vi "Parse Floating Point String As Extended.vi"(8 "error in (no error)":errorcluster, 11 "String":string) -> (0 "error out":errorcluster, 3 "Value":variant)   [LabVIEW 2019, in "JKI JSON Serialization.lvlib" / "JSON Parser.lvclass"]
doc: "JKI JSON 1.1.10.37\nTomi Maila - JKI\nCopyright (c) 2017, JKI"
uses:
  JSON Parser.lvclass
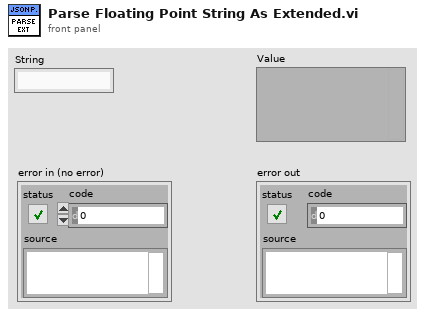
[diagram p1: front panel]
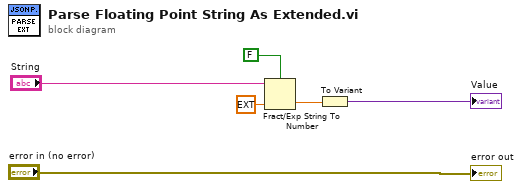
[diagram p0: block diagram]
diagram:
  n1 = Fract/Exp String To Number(use system decimal point (T)=FALSE, string="String", default (0 dbl)=ext 0.0 ("default (0 I32)")) -> (number=w2:ext)  [unwired: 1 in, 1 out]
  n2 = To Variant(anything=w2) -> (Variant=→"Value":variant)
  "error out" <- "error in (no error)"
